vi "test1.vi"() -> ()   [LabVIEW 2022 SP3]
panel:
  in  "stop":bool
  out "data":dbl
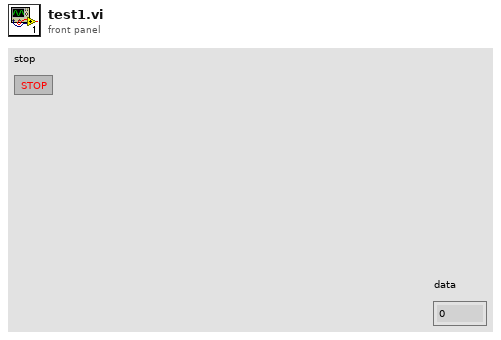
[diagram p1: front panel]
types:
  T1 = enum32{"Invalid", "Standard", "Closed", "Hidden", "Minimized", "Maximized"}
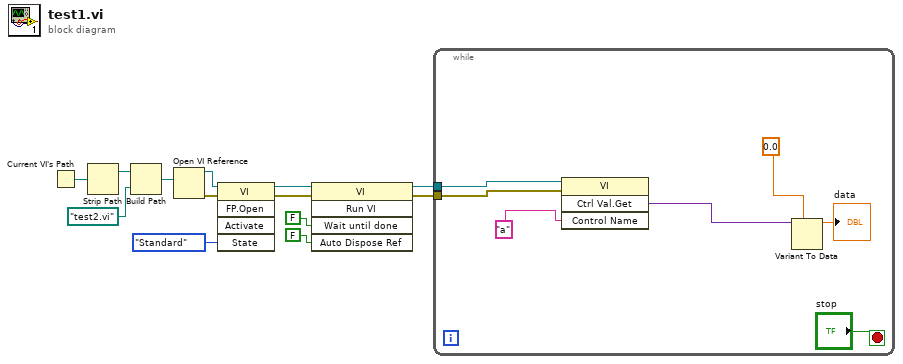
[diagram p0: block diagram]
diagram:
  n1 = Current VI's Path() -> (path=w13:path)
  n2 = Strip Path(path=w13) -> (stripped path=w12:path)  [unwired: 1 out]
  n3 = Build Path(base path=w12, name or relative path=path "test2.vi") -> (appended path=w10:path)
  n4 = Open VI Reference(vi path=w10) -> (vi reference=w9:refnum<vi>, error out=w7:errorcluster)  [unwired: 5 in]
  n5 = invoke class="VI" method="FP.Open"(reference=w9, error in=w7, "State"=T1."Standard") -> (reference out=w4:refnum<vi>, error out=w3:errorcluster)  [unwired: 2 in, 3 out]
  n6 = invoke class="VI" method="Run VI"(reference=w4, error in=w3, "Wait until done"=FALSE ("Wait Until Done"), "Auto Dispose Ref"=FALSE ("Auto Dispose Reference")) -> (reference out=w2:refnum<vi>, error out=w1:errorcluster)  [unwired: 1 in, 3 out]
  n7 = while {
    tunnel: w2 -> [w20]
    tunnel: w1 -> [w19]
    stop <- "stop" stop-if-true
    n8 = invoke class="VI" method="Ctrl Val.Get"(reference=w20, error in=w19, "Control Name"="a") -> ("Get Control Value Variant"=w17:variant)  [unwired: 1 in, 3 out]
    n9 = Variant To Data(type=0.0, Variant=w17) -> (data=→"data":dbl)  [unwired: 1 in, 1 out]
  }
